vi "Carro instrumentacion Jorge Parra.vi"() -> ()   [LabVIEW 2024]
panel:
  in  "Velocidad":dbl(slide) scale=0.0..5.0
  in  "Freno":dbl(slide) scale=0.0..5.0
  in  "Acelerar":dbl(slide) scale=0.0..3.0
  out "Temperatura":dbl(knob) scale=0.0..10.0
  out "Tacometro":dbl(knob) scale=0.0..5.0
  out "Velocimetro":dbl(knob) scale=0.0..200.0
  out "Inter 2":bool
  out "Inter 1":bool
  out "Derecha":bool
  out "Izquierda":bool
  in  "Intermitentes":bool
  in  "Llenar Tanque":bool
  in  "stop":bool
  in  "Derecha":bool
  in  "Izquierda":bool
  out "GAS":dbl(knob) scale=0.0..10.0
  in  "Encender/apagar":bool
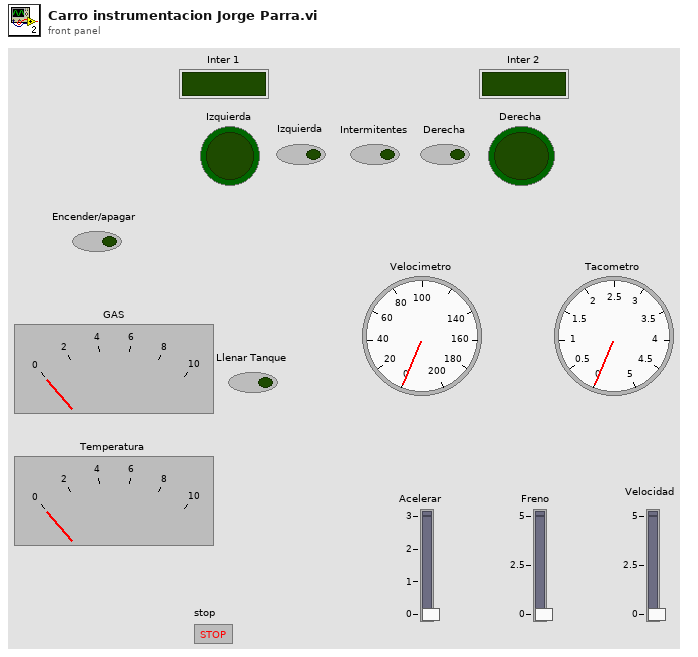
[diagram p1: front panel]
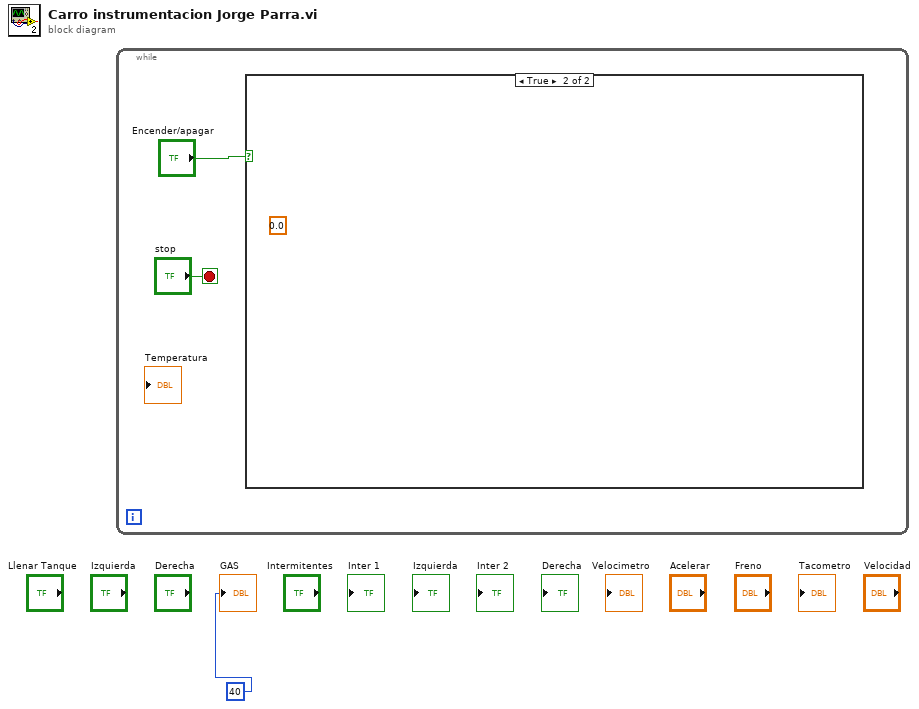
[diagram p0: block diagram]
diagram:
  n1 = while {
    stop <- "stop" stop-if-true
    n2 = case shown="True" "Encender/apagar" {
      frame False {
      }
      frame True {
        (unwired) 0.0
      }
    }
  }
  "GAS" <- 40
